vi "Launch Associated GUI.vi"(8 "error in (no error)":errorcluster, 10 "GUI Class":string, 11 "CS++BaseActor in":refnum<class "CS++BaseActor.lvclass">) -> (0 "error out":errorcluster, 3 "CS++BaseActor out":refnum<class "CS++BaseActor.lvclass">)   [LabVIEW 2015, in "CS++BaseActor.lvlib" / "CS++BaseActor.lvclass"]
doc: "Launch Associated GUI for this actor."
uses:
  CS++BaseActor.lvclass
  CS++BaseActor.lvclass/CS++BaseActor.ctl
  <vilib>/ActorFramework/Actor/Actor.lvclass/Actor.ctl
  <vilib>/ActorFramework/Message Enqueuer/Message Enqueuer.lvclass/Message Enqueuer.ctl
  CS++GUIActor/CS++GUIActor.lvclass
  CS++PVProxy/CS++PVProxy.lvclass
  CS++GUIActor/CS++GUIActor.lvclass/CS++GUIActor.ctl
  CS++BaseActor Messages/Open Actor Core FP Msg/Open Actor Core FP Msg.lvclass/Open Actor Core FP Msg.ctl
  <vilib>/ActorFramework/Message Enqueuer/Init from Existing Queue.vi
  <vilib>/ActorFramework/Message Enqueuer/Enqueue.vi
  <vilib>/ActorFramework/Message Priority Queue/Priority Enqueue.vi
  CS++BaseActor Messages/Open Actor Core FP Msg/Open Actor Core FP Msg.lvclass
  <vilib>/ActorFramework/Message Enqueuer/Message Enqueuer.lvclass
  Classes/CS++BaseClasses/Factory/CS++Factory.lvclass
  <vilib>/ActorFramework/Actor/Actor.lvclass
  Libraries/Utilities/CS++Utilities.lvlib
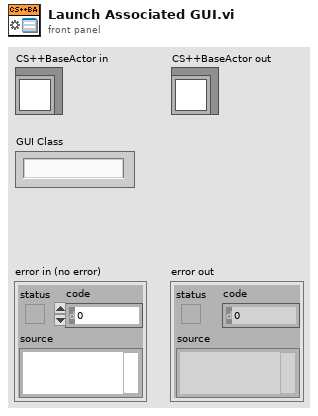
[diagram p1: front panel]
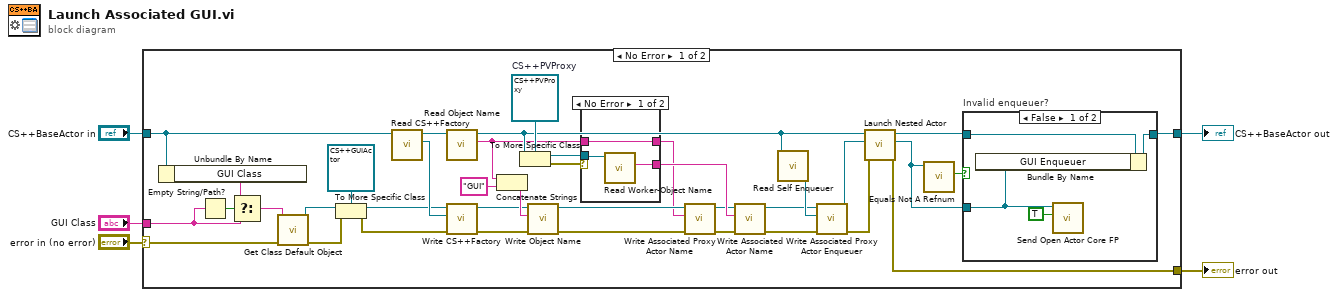
[diagram p0: block diagram]
diagram:
  n1 = case shown="No Error" "error in (no error)" {
    selector: "error in (no error)" -> [w23 w54]
    tunnel: [w27 w54] -> w4
    tunnel: [w39 w53] -> w2
    tunnel: "CS++BaseActor in" -> [w34 w53]
    tunnel: "GUI Class" -> [w41 _]
    frame No Error {
      w18 = refnum<class "CS++PVProxy.lvclass"> refnum  # CS++PVProxy
      n2 = Unbundle By Name(w34) -> ("GUI Class"=w42:string)
      n3 = Empty String/Path?(string/path=w41) -> (empty?=w43:bool)
      n4 = Select(t=w42, s=w43, f=w41) -> (s? t:f=w24:string)
      n5 = call "Get Class Default Object.vi"("Error In"=w23, "Class"=w24) -> ("Error Out"=w22:errorcluster, "Class Default Object"=w21:refnum<class>)  [unwired: 8 in]
      n6 = To More Specific Class(target class=refnum<class "CS++GUIActor.lvclass"> refnum ("CS++DeviceGUIActor.lvlib:CS++DeviceGUIActor.lvclass"), reference=w21, error in=w22) -> (specific class reference=w20:refnum<class "CS++GUIActor.lvclass">, error out=w19:errorcluster)
      n7 = call "Read CS++Factory.vi"("CS++BaseActor in"=w34) -> ("CS++Factory"=w30:refnum<class "CS++Factory.lvclass">, "CS++BaseActor out"=w33:refnum<class "CS++BaseActor.lvclass">)  [unwired: 8 in, 1 out]
      n8 = call "Read Object Name.vi"("CS++BaseActor in"=w33) -> ("Object Name"=w9:string, "CS++BaseActor out"=w11:refnum<class "CS++BaseActor.lvclass">)  [unwired: 8 in, 1 out]
      n9 = call "Write CS++Factory.vi"("error in (no error)"=w19, "CS++Factory"=w30, "CS++BaseActor in"=w20) -> ("error out"=w31:errorcluster, "CS++BaseActor out"=w32:refnum<class "CS++GUIActor.lvclass">)  [unwired: 7 in]
      n10 = Concatenate Strings(w9, "GUI" ("string")) -> (w35:string)
      n11 = To More Specific Class(target class=w18, reference=w11) -> (specific class reference=w12:refnum<class "CS++PVProxy.lvclass">, error out=w6:errorcluster)  [unwired: 1 in]
      n12 = call "Write Object Name.vi"("error in (no error)"=w31, "Object Name"=w35, "CS++BaseActor in"=w32) -> ("error out"=w13:errorcluster, "CS++BaseActor out"=w14:refnum<class "CS++GUIActor.lvclass">)  [unwired: 7 in]
      n13 = case shown="No Error" w6 {
        tunnel: w12 -> [w46 _]
        tunnel: [w45 w47] -> w17
        tunnel: [w44 _] -> w10
        tunnel: w9 -> [w44 w47]
        frame No Error {
          n14 = call-dynamic "Read Worker-Object Name.vi"("CS++PVProxy in"=w46) -> ("Worker-Object Name"=w45:string)  [unwired: 8 in, 2 out]
        }
        frame Error {
        }
      }
      n15 = call "Write Associated Proxy Actor Name.vi"("error in (no error)"=w13, "Associated Proxy Actor Name"=w10, "CS++GUIActor in"=w14) -> ("error out"=w7:errorcluster, "CS++GUIActor out"=w8:refnum<class "CS++GUIActor.lvclass">)  [unwired: 7 in]
      n16 = call "Write Associated Actor Name.vi"("error in (no error)"=w7, "Associated Actor Name"=w17, "CS++GUIActor in"=w8) -> ("error out"=w15:errorcluster, "CS++GUIActor out"=w16:refnum<class "CS++GUIActor.lvclass">)  [unwired: 7 in]
      n17 = call <vilib>:"Read Self Enqueuer.vi"("Actor"=w11) -> ("Self Enqueuer"=w37:refnum<class "Message Enqueuer.lvclass">)  [unwired: 10 in]
      n18 = call "Write Associated Proxy Actor Enqueuer.vi"("error in (no error)"=w15, "Actor Framework:Message Enqueuer"=w37, "CS++GUIActor in"=w16) -> ("error out"=w26:errorcluster, "CS++GUIActor out"=w25:refnum<class "CS++GUIActor.lvclass">)  [unwired: 7 in]
      n19 = call <vilib>:"Launch Nested Actor.vi"("error in (no error)"=w26, "Nested Actor"=w25, "Caller Actor in"=w11) -> ("error out"=w27:errorcluster, "Nested Actor's Enqueuer"=w28:refnum<class "Message Enqueuer.lvclass">, "Caller Actor out"=w29:refnum<class "CS++BaseActor.lvclass">)  [unwired: 6 in]
      n20 = call <vilib>:"Equals Not A Refnum.vi"("Message Enqueuer"=w28) -> ("Not a refnum?"=w38:bool)  [unwired: 10 in]
      n21 = case "Invalid enqueuer?" shown="False" w38 {
        tunnel: w29 -> [w51 w52]
        tunnel: [w50 w52] -> w39
        tunnel: w28 -> [w49 _]
        frame False {
          n22 = Bundle By Name(cluster=w51, "GUI Enqueuer"=w49) -> (w50:refnum<class "CS++BaseActor.lvclass">)
          n23 = call "Send Open Actor Core FP.vi"("Open FP (F)"=TRUE, "Message Enqueuer"=w49) -> ()  [unwired: 8 in, 2 out]
        }
        frame True {
        }
      }
    }
    frame Error {
    }
  }
  "error out" <- w4
  "CS++BaseActor out" <- w2
